vi "set_trigger.vi"() -> ()   [LabVIEW 2020]
panel:
  out "display file":string
  in  "Path":path
  out "display m3510A":string
  in  "Voltmeter Picotest M3510A":refnum<visa-resource-name>
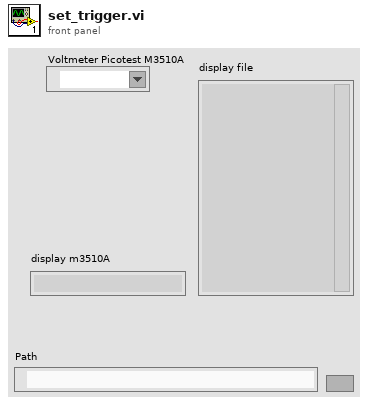
[diagram p1: front panel]
types:
  T1 = enum16{"read/write", "read-only", "write-only", ""}
  T2 = enum16{"open", "replace", "create", "open or create", "replace or create", "replace or create with confirmation", ""}
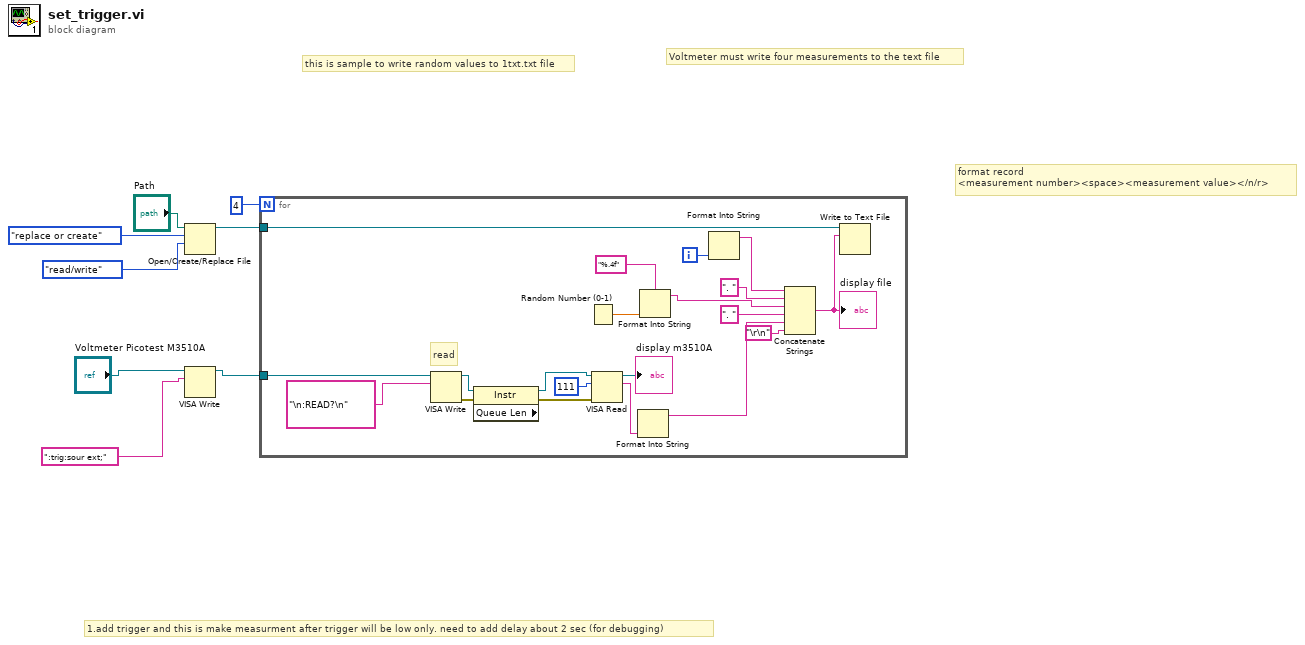
[diagram p0: block diagram]
diagram:
  # "1.add trigger and this is make measurment after trigger will be low only. need to add delay about 2 sec (for debugging)"
  # "format record \n<measurement number><space><measurement value></n/r>"
  # "Voltmeter must write four measurements to the text file"
  # "this is sample to write random values to 1txt.txt file"
  n1 = Open/Create/Replace File(file path (use dialog)="Path", operation (0:open)=T2."replace or create", access (0:read/write)=T1."read/write") -> (refnum out=w4:refnum<file>)  [unwired: 3 in, 2 out]
  n2 = VISA Write(VISA resource name="Voltmeter Picotest M3510A", write buffer=":trig:sour ext;") -> (VISA resource name out=w3:refnum<visa-resource-name>)  [unwired: 1 in, 2 out]
  n3 = for {
    N: 4 -> [_]
    tunnel: w3 -> [w12]
    tunnel: w4 -> [w10]
    i -> [w22]
    # "read"
    n4 = VISA Write(VISA resource name=w12, write buffer="\n:READ?\n") -> (VISA resource name out=w26:refnum<visa-resource-name>, error out=w27:errorcluster)  [unwired: 1 in, 1 out]
    n5 = property class="Instr" props=["Queue Len"](reference=w26, error in=w27) -> (reference out=w25:refnum<visa-resource-name>, error out=w24:errorcluster)  [unwired: 1 out]
    n6 = Random Number (0-1)() -> (number: 0 to 1=w23:dbl)
    n7 = VISA Read(VISA resource name=w25, byte count=111, error in (no error)=w24) -> (VISA resource name out=→"display m3510A":refnum<visa-resource-name>, read buffer=w13:string)  [unwired: 2 out]
    n8 = Format Into String(w13) -> (resulting string=w15:string)  [unwired: 3 in, 1 out]
    n9 = Format Into String(format string="%.4f", w23) -> (resulting string=w19:string)  [unwired: 2 in, 1 out]
    n10 = Format Into String(w22) -> (resulting string=w21:string)  [unwired: 3 in, 1 out]
    n11 = Concatenate Strings(w21, ". ", w19, ". ", w15, "\r\n") -> (w11:string)
    "display file" <- w11
    n12 = Write to Text File(file (use dialog)=w10, text=w11) -> ()  [unwired: 2 in, 3 out]
  }
